vi "S7COMM - Build Params - any-type Addressing.vi"(4 "Start Address":T2, 5 "Bit Offset":u8, 6 "S7_Memory_Area":T3 items=["P Area"=128, "I Area"=129, "O Area"=130, "M Area"=131, "DB Area"=132, "Counter"=40, "Timer"=41], 7 "S7_Function_Code":T1 items=["Read"=4, "Write"=5], 8 "Item Count":u8=1, 9 "DB Number":u16, 10 "Count":u16, 11 "S7_Variable_Type":T4=enum."BIT") -> (3 "S7 Params Byte Array":T5 format="0x%02x")   [LabVIEW 2014, in "S7NetCom.lvclass"]
doc: "____\nCopyright (c) 2019 Hampel Software Engineering (HSE), released under BSD license. More info can be found on https://dokuwiki.hampel-soft.com/code/hse/s7netcom. Original code published by Marc Christenson, Sisu Devices."
uses:
  S7NetCom.lvclass
  Controls/S7NetCom_HexByteArray.ctl
  Controls/S7NetCom_HexByte.ctl
  Controls/S7_Variable_Type.ctl
  Controls/S7_Memory_Area.ctl
  Controls/S7_Start_Address.ctl
  S7COMM - Function Codes--ring.ctl
panel:
  # "More info on https://dokuwiki.hampel-soft.com/code/hse/s7netcom\n\nCopyright (c) 2019, HAMPEL SOFTWARE ENGINEERING (HSE)\nOriginal code developed by Marc Christenson, Sisu Devices\nAll rights reserved.\n\nRedistribution and use in source and binary forms, with or without\nmodification, are permitted provided that the following conditions are met:\n\n1. Redistributions of source code must retain the above copyright\n   notice, this list of conditions and the following disclaimer.\n\n2. Redistributions in binary form must reproduce the above copyright\n   notice, this list of conditions and the following disclaimer in the\n   documentation and/or other materials provided with the distribution.\n\n3. All advertising materials mentioning features or use of this software\n   must display the following acknowledgement:\n   This product includes software developed by HAMPEL SOFTWARE ENGINEERING.\n\n4. Neither the name of HAMPEL SOFTWARE ENGINEERING nor the\n   names of its contributors may be used to endorse or promote products\n   derived from this software without specific prior written permission.\n\nTHIS SOFTWARE IS PROVIDED BY HAMPEL SOFTWARE ENGINEERING ''AS IS'' AND ANY\nEXPRESS OR IMPLIED WARRANTIES, INCLUDING, BUT NOT LIMITED TO, THE IMPLIED\nWARRANTIES OF MERCHANTABILITY AND FITNESS FOR A PARTICULAR PURPOSE ARE\nDISCLAIMED. IN NO EVENT SHALL HAMPEL SOFTWARE ENGINEERING BE LIABLE FOR ANY\nDIRECT, INDIRECT, INCIDENTAL, SPECIAL, EXEMPLARY, OR CONSEQUENTIAL DAMAGES\n(INCLUDING, BUT NOT LIMITED TO, PROCUREMENT OF SUBSTITUTE GOODS OR SERVICES;\nLOSS OF USE, DATA, OR PROFITS; OR BUSINESS INTERRUPTION) HOWEVER CAUSED AND\nON ANY THEORY OF LIABILITY, WHETHER IN CONTRACT, STRICT LIABILITY, OR TORT\n(INCLUDING NEGLIGENCE OR OTHERWISE) ARISING IN ANY WAY OUT OF THE USE OF THIS\nSOFTWARE, EVEN IF ADVISED OF THE POSSIBILITY OF SUCH DAMAGE."
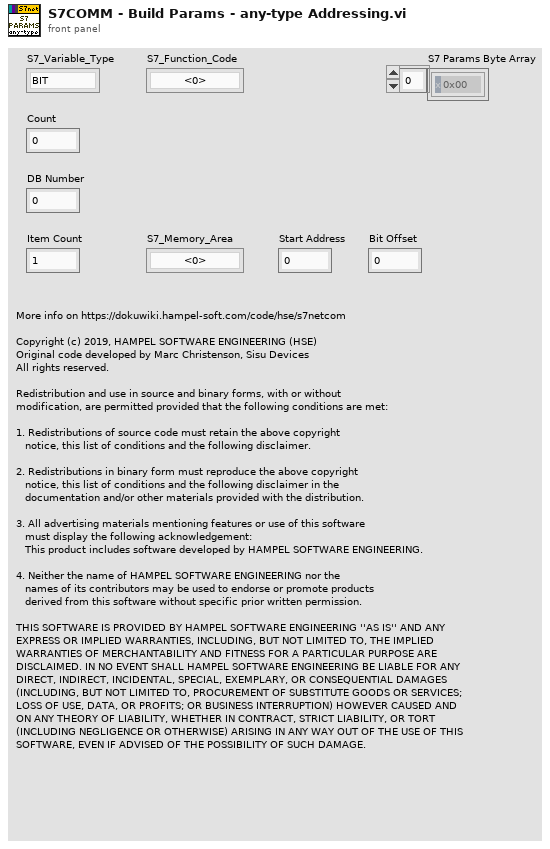
[diagram p1: front panel]
types:
  T1 = typedef "S7NetCom.lvclass/S7COMM - Function Codes--ring.ctl" = u8
  T2 = typedef "S7NetCom.lvclass/S7_Start_Address.ctl" = u32
  T3 = typedef "S7NetCom.lvclass/S7_Memory_Area.ctl" = u8
  T4 = typedef "S7NetCom.lvclass/S7_Variable_Type.ctl" = enum8{"---", "BIT", "BYTE", "CHAR", "WORD", "INT", "DWORD", "DINT", "REAL"}
  T5 = typedef "S7NetCom.lvclass/S7NetCom_HexByteArray.ctl" = T6[]
  T6 = typedef "S7NetCom.lvclass/S7NetCom_HexByte.ctl" = u8
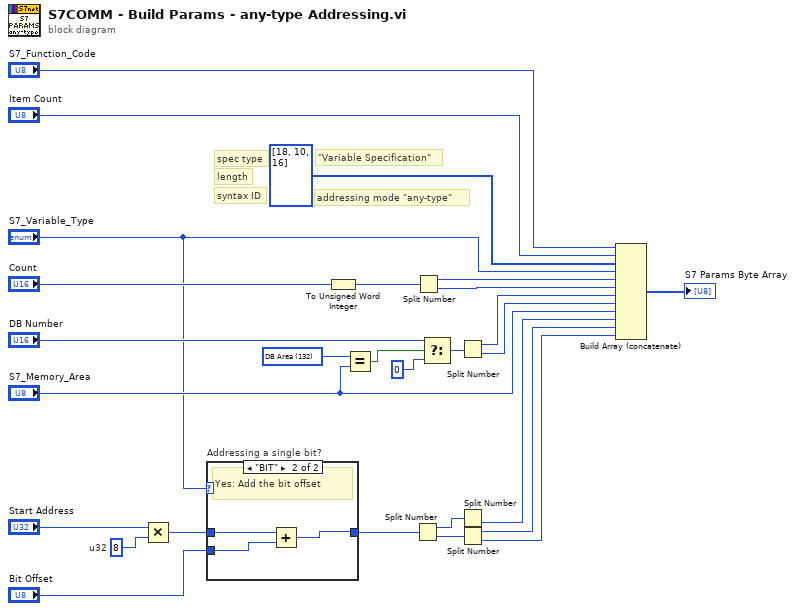
[diagram p0: block diagram]
diagram:
  w23 = T3 132 items=["P Area"=128, "I Area"=129, "O Area"=130, "M Area"=131, "DB Area"=132, "Counter"=40, "Timer"=41] ("S7_Address_Area")
  w13 = T2 8  # u32
  # "addressing mode \"any-type\""
  # "\"Variable Specification\""
  # "spec type"
  # "length"
  # "syntax ID"
  n1 = Multiply(x="Start Address", y=w13) -> (x*y=w3:T2)
  n2 = case "Addressing a single bit?" shown="\"BIT\"" "S7_Variable_Type" {
    tunnel: w3 -> [w28 w31]
    tunnel: [w28 w30] -> w1
    tunnel: "Bit Offset" -> [_ w29]
    frame "---", Default {
      # "No: Do nothing"
    }
    frame "BIT" {
      # "Yes: Add the bit offset"
      n3 = Add(x=w31, y=w29) -> (x+y=w30:T2)
    }
  }
  n4 = To Unsigned Word Integer(number="Count") -> (unsigned 16bit integer=w22:u16)
  n5 = Equal?(x=w23, y="S7_Memory_Area") -> (x = y?=w12:bool)
  n6 = Split Number(x=w1) -> (hi(x)=w14:u16, lo(x)=w15:u16)
  n7 = Split Number(x=w22) -> (hi(x)=w18:u8, lo(x)=w17:u8)
  n8 = Select(t="DB Number", s=w12, f=u16 0) -> (s? t:f=w9:u16)
  n9 = Split Number(x=w9) -> (hi(x)=w10:u8, lo(x)=w11:u8)
  n10 = Split Number(x=w14) -> (lo(x)=w21:u8)  [unwired: 1 out]
  n11 = Split Number(x=w15) -> (hi(x)=w20:u8, lo(x)=w19:u8)
  n12 = Build Array (concatenate)("S7_Function_Code", "Item Count", u8[] [18, 10, 16] ("Item Count, Item Header"), "S7_Variable_Type", w18, w17, w10, w11, "S7_Memory_Area", w21, w20, w19) -> (→"S7 Params Byte Array":T3[])
